vi "Easy XML Editor.vi"() -> ()   [LabVIEW 2026, in "VILab.lvlib"]
doc: "A tool for editing LabVIEW objects as XML that's quicker than using the other resource editor VI."
uses:
  VILab.lvlib
  CTLs/XML Editor State Data.ctl
  CTLs/Resource.ctl
  <vilib>/Utility/miscctls.llb/LVPositionTypeDef.ctl
  <vilib>/ErrorRing/Error Ring.xnode
  SubVIs/FaKI State Machine/FaKI State Machine.lvlib
panel:
  in  "Exit":bool
  in  "Paste FP":bool
  in  "Copy FP":bool
  in  "Front Panel XML/VTT":string
  in  "Paste BD":bool
  in  "Copy BD":bool
  in  "Block Diagram XML/VTT":string
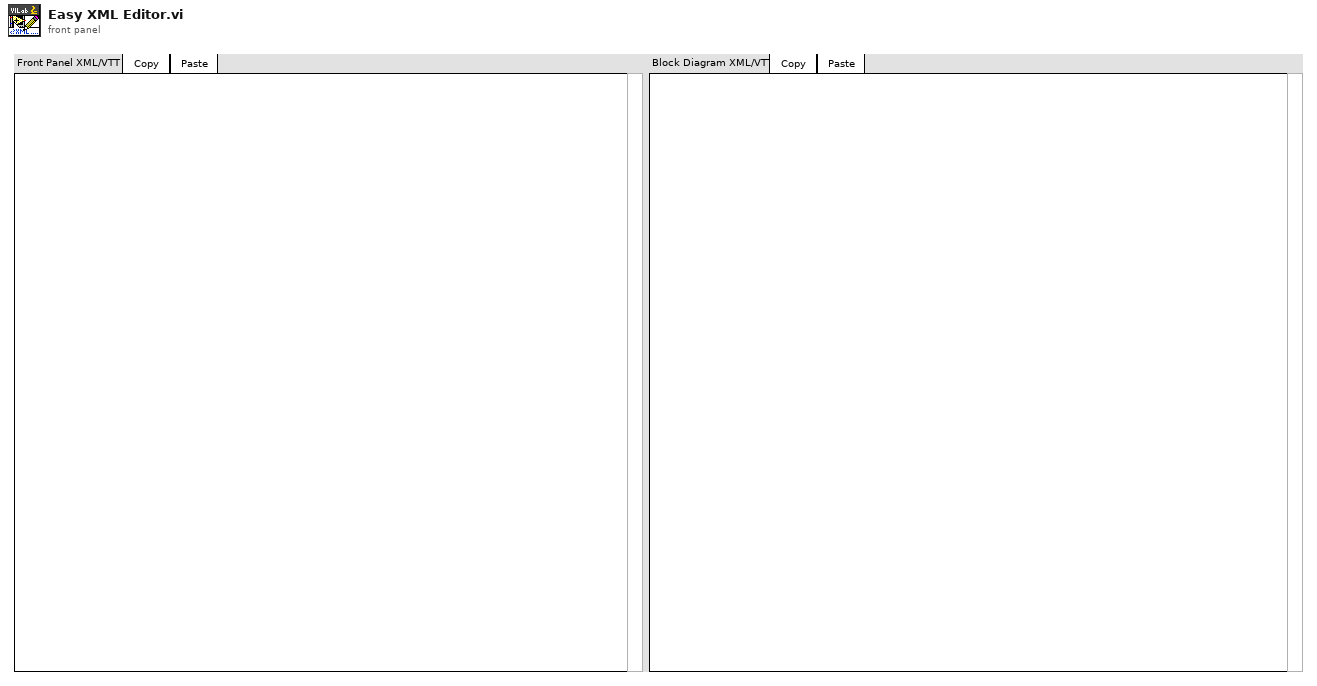
[diagram p1: front panel]
types:
  T1 = typedef "VILab.lvlib/XML Editor State Data.ctl" = cluster{"Core":cluster{"Current VI Ref":refnum<vi>, "Close Panel on Exit?":bool, "Menu Ref":refnum<k9>}, "Stored Resources":T2[], "Use Stored Resources?":bool, "Last Edited VI Path":path, "Use VTT?":bool, "Source VI Ref":refnum<vi>, "Booleans":cluster{"Refnum":refnum<vi>, "Position":T3}[], "FP XML":string, "BD XML":string}
  T2 = typedef "VILab.lvlib/Resource.ctl" = cluster{"type":u32, "id":i32, "name":string, "binary data":string}
  T3 = typedef "LVPositionTypeDef.ctl" = cluster{"Left":i32, "Top":i32}
  T4 = enum32{"Invalid", "Standard", "Closed", "Hidden", "Minimized", "Maximized"}
  T5 = enum32{"invalid app kind", "Development System", "Run Time System", "Student Edition", "Embedded LabVIEW", "Evaluation", "Custom"}
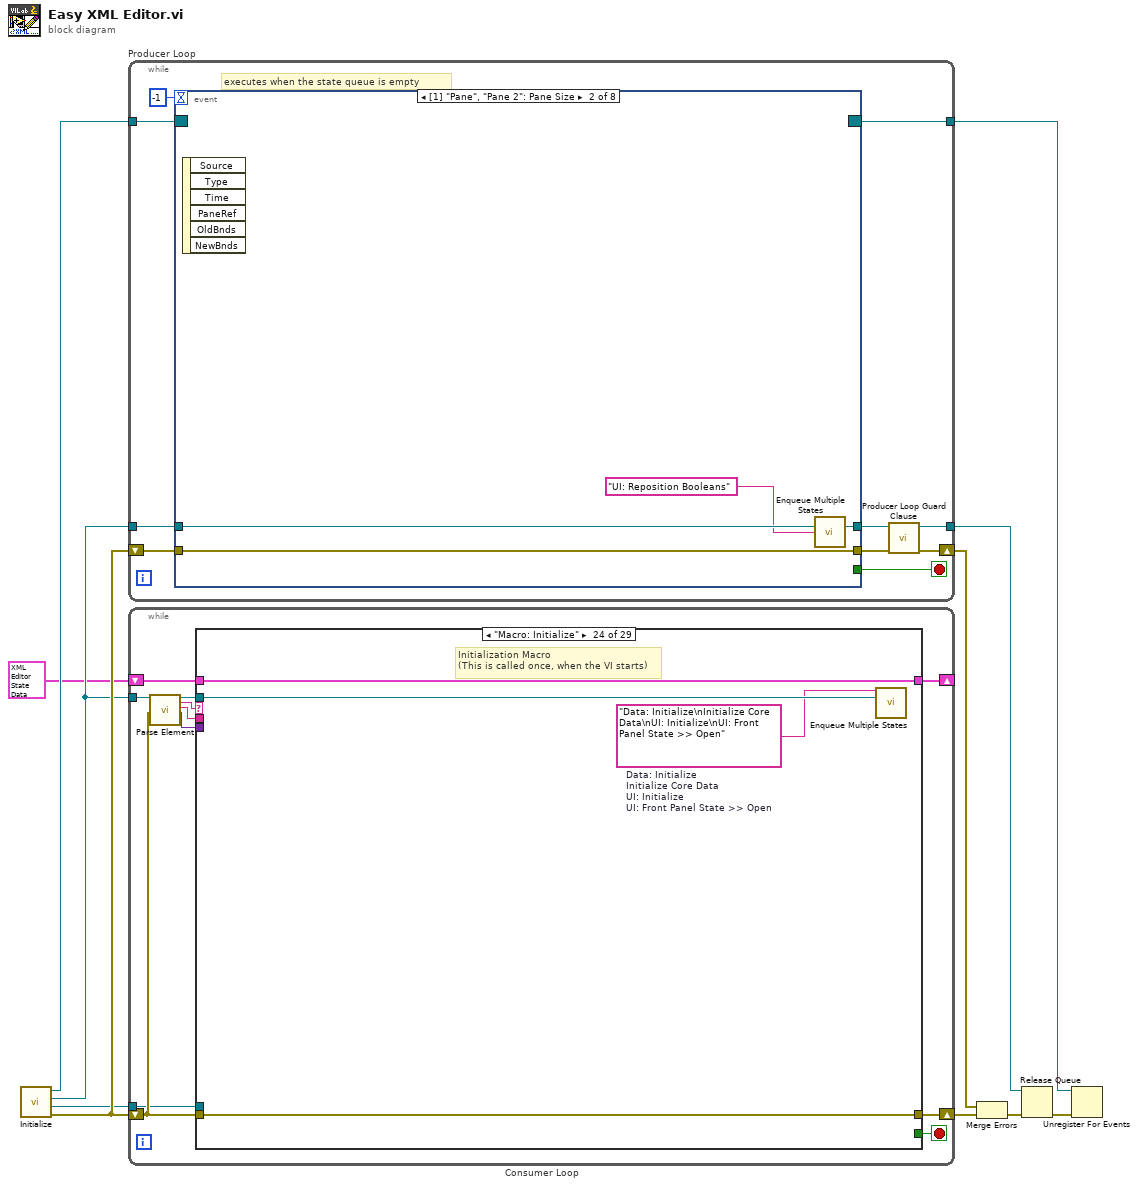
[diagram p0: block diagram]
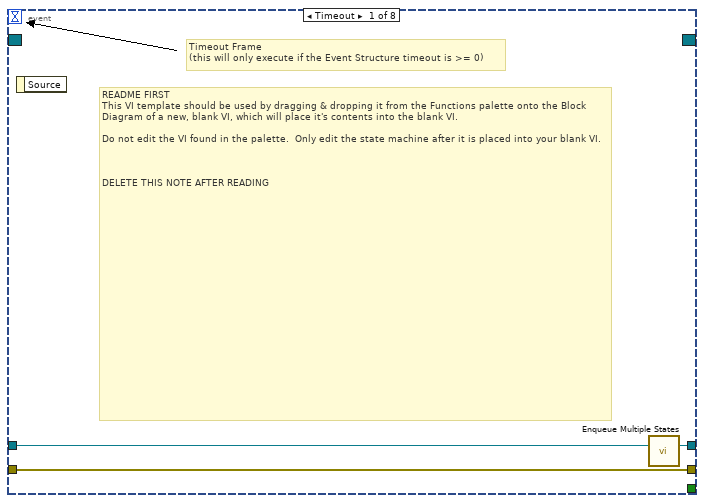
[diagram p2: hidden frame]
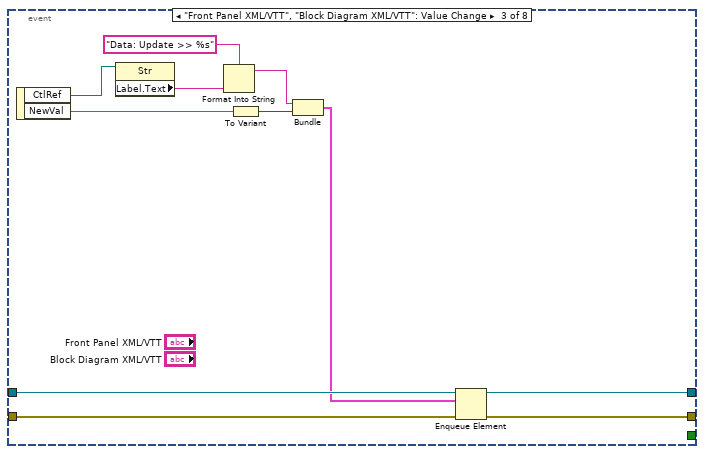
[diagram p3: hidden frame]
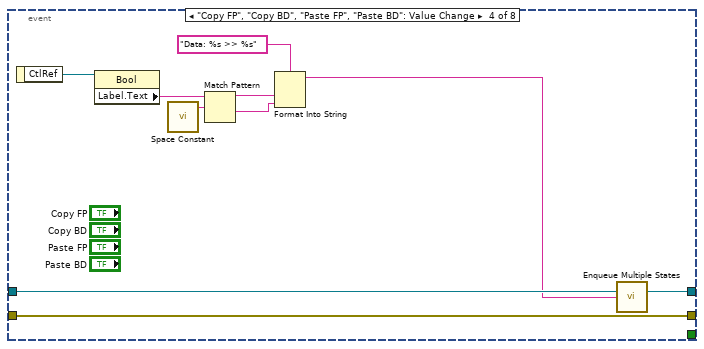
[diagram p4: hidden frame]
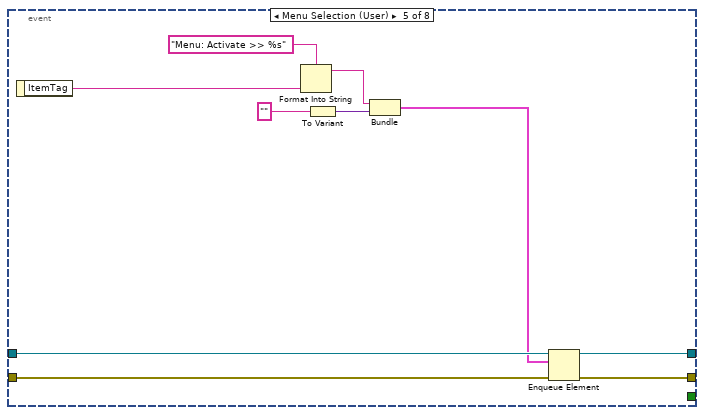
[diagram p5: hidden frame]
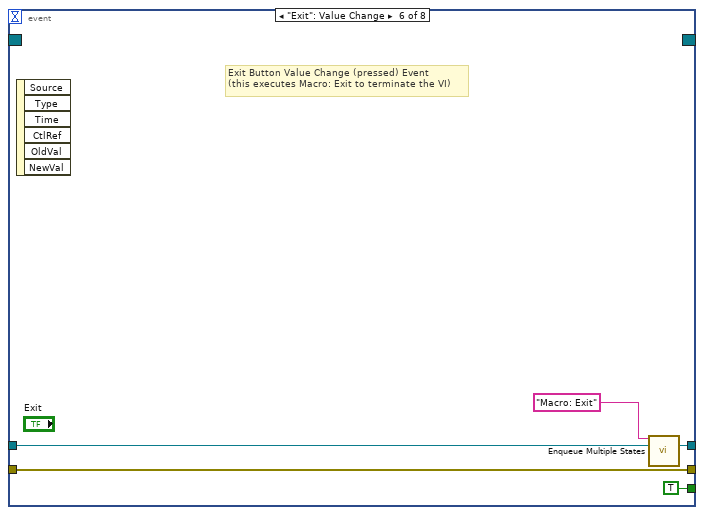
[diagram p6: hidden frame]
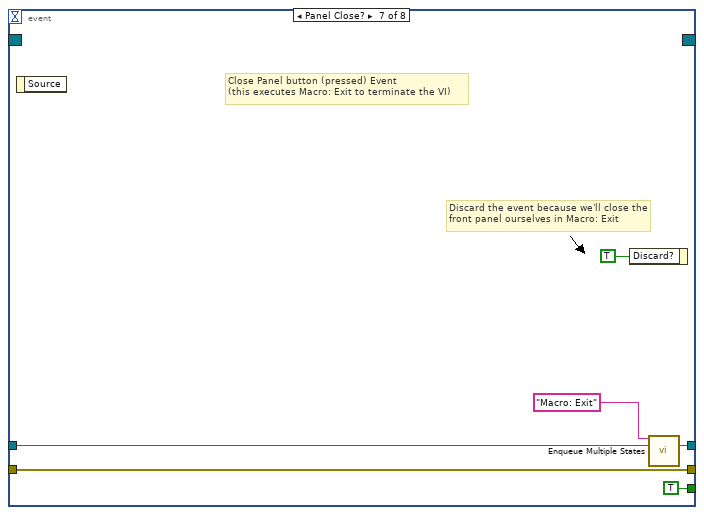
[diagram p7: hidden frame]
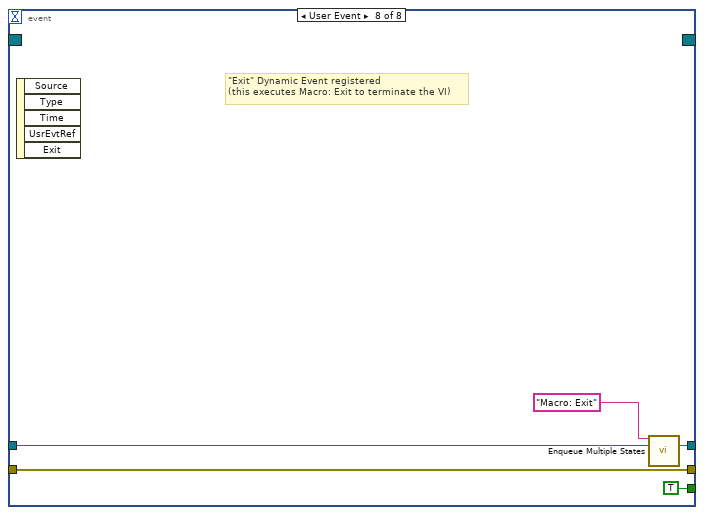
[diagram p8: hidden frame]
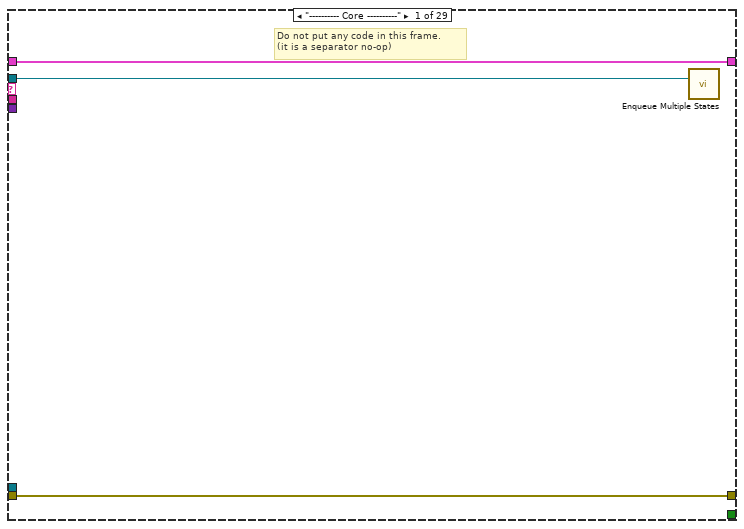
[diagram p9: hidden frame]
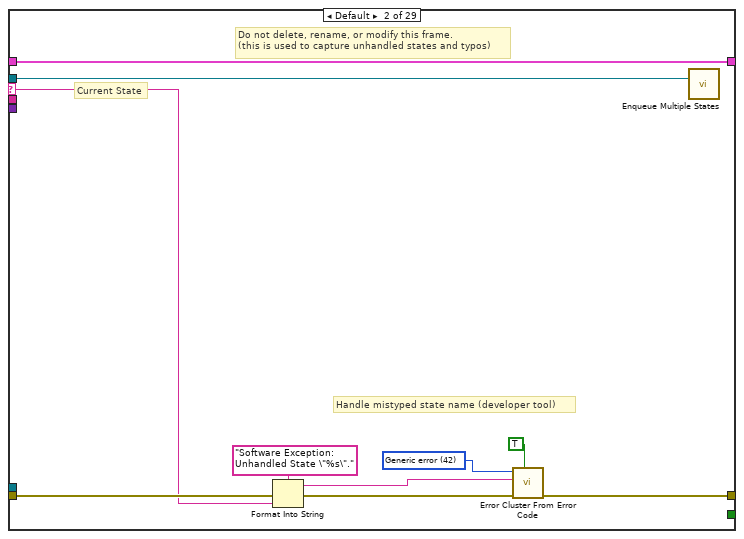
[diagram p10: hidden frame]
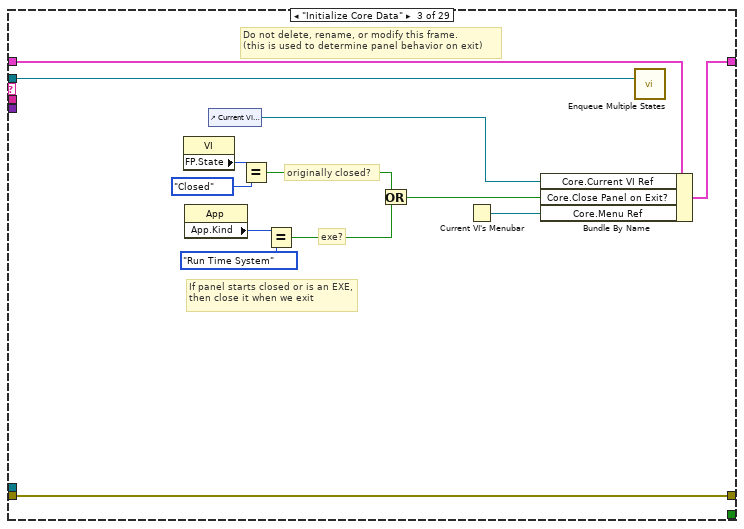
[diagram p11: hidden frame]
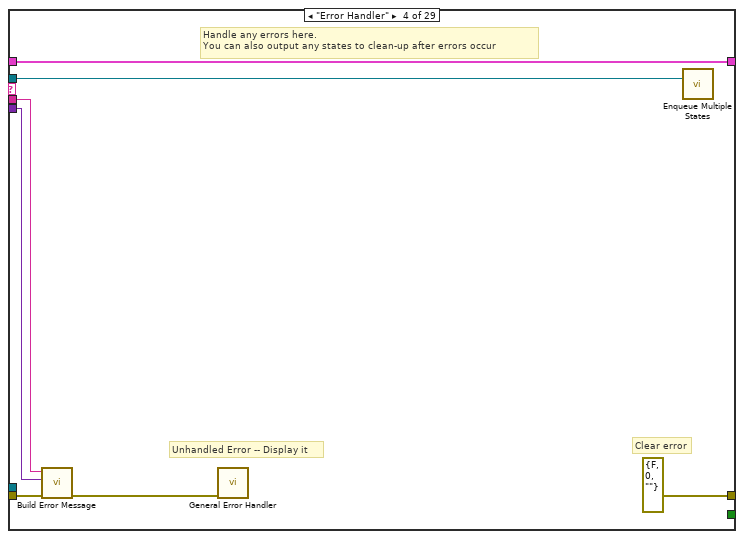
[diagram p12: hidden frame]
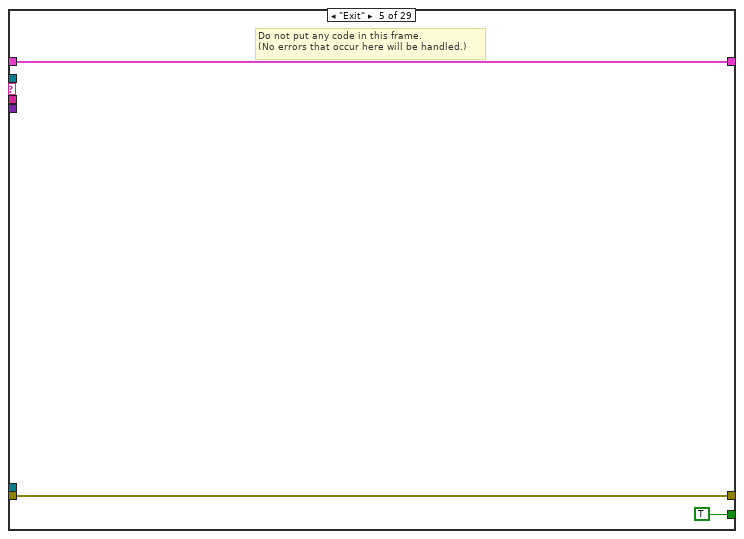
[diagram p13: hidden frame]
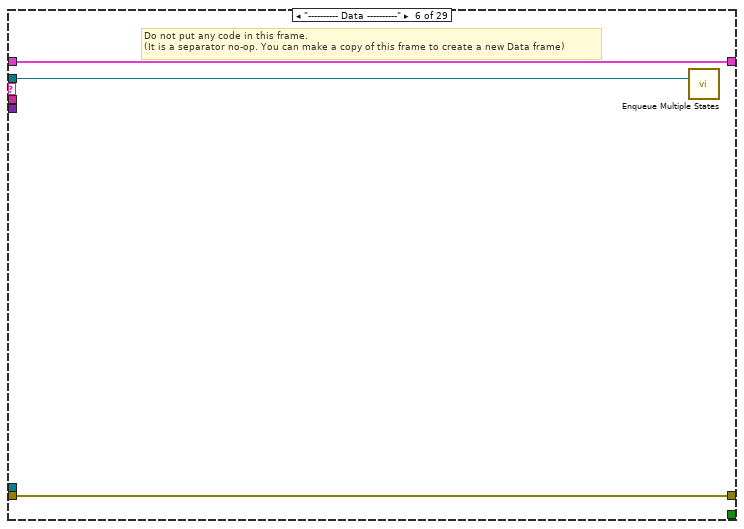
[diagram p14: hidden frame]
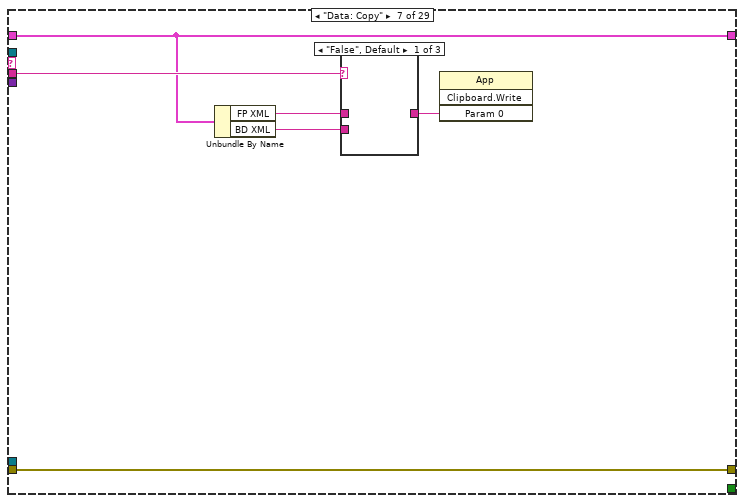
[diagram p15: hidden frame]
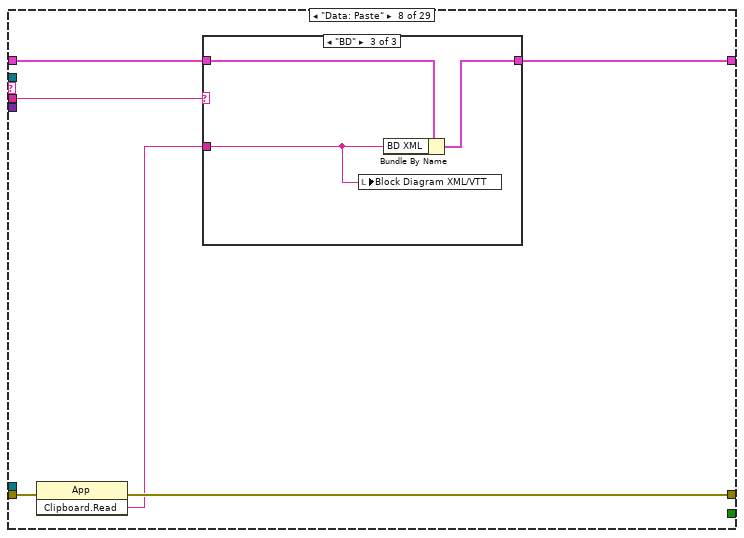
[diagram p18: hidden frame]
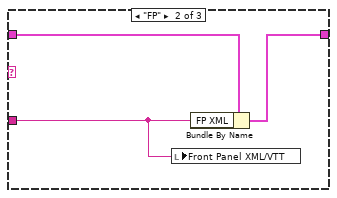
[diagram p20: hidden frame]
diagram:
  n1 = call "Initialize.vi"() -> ("error out"=w7:errorcluster, "Exit Event out"=w4:refnum<user-event>, "queue out"=w6:refnum<queue>, "Event Registration Refnum out"=w5:refnum<event-registration>)  [unwired: 8 in]
  n2 = while "Producer Loop" {
    shift-right: [w16] -> w10
    shift-left: w7 -> [w21]
    tunnel: w5 -> [w13]
    tunnel: w6 -> [w19]
    tunnel: [w14] -> w8
    tunnel: [w12] -> w2
    stop <- w18 stop-if-true
    # "executes when the state queue is empty"
    n3 = event shown="[1] \"Pane\", \"Pane 2\": Pane Size" {
      selector: w13 -> [_ _ _ _ _ _ _ _]
      dyn-events: [_ _ _ _ _ _ _ _] -> w12
      timeout: -1 ("Timeout") -> [_ _ _ _ _ _ _ _]
      tunnel: [w22 w26 w38 w49 w58 w64 w70 w75] -> w17
      tunnel: w21 -> [w22 w26 w39 w49 w59 w64 w70 w75]
      tunnel: w19 -> [w23 w27 w37 w48 w57 w63 w67 w73]
      tunnel: [w24 w28 w36 w47 w56 w61 w66 w72] -> w15
      tunnel: [_ _ _ _ _ TRUE TRUE TRUE] -> w18
      event Timeout {
        # "README FIRST\nThis VI template should be used by dragging & dropping it from the Functions palette onto the Block Diagram of a new, blank VI, which will place it's contents into the blank VI.\n\nDo not edit the VI found in the palette.  Only edit the state machine after it is placed into your blank VI.\n\n\n\nDELETE THIS NOTE AFTER READING"
        # "Timeout Frame\n(this will only execute if the Event Structure timeout is >= 0)"
        n4 = event-data() -> ()  [unwired: 1 in, 1 out]
        n5 = call "Enqueue Multiple States.vi"("queue in"=w23) -> ("queue out"=w24:refnum<queue>)  [unwired: 14 in]
      }
      event Pane Size {
        n6 = event-data() -> ()  [unwired: 1 in, 6 out]
        n7 = call "Enqueue Multiple States.vi"("queue in"=w27, "State(s) at Back"="UI: Reposition Booleans") -> ("queue out"=w28:refnum<queue>)  [unwired: 13 in]
      }
      event "Front Panel XML/VTT", "Block Diagram XML/VTT": Value Change {
        n8 = event-data() -> ("CtlRef"=w35:refnum<vi>, "NewVal"=w32:string)  [unwired: 1 in]
        n9 = property class="Str"(reference=w35) -> ("Label.Text"=w33:string)  [unwired: 1 in, 2 out]
        n10 = Format Into String(format string="Data: Update >> %s", w33) -> (resulting string=w30:string)  [unwired: 2 in, 1 out]
        n11 = To Variant(anything=w32) -> (Variant=w31:variant)
        n12 = Bundle(w30, "Variant"=w31) -> (w29:cluster{string, "Variant":variant})  [unwired: 1 in]
        n13 = Enqueue Element(queue=w37, element=w29, error in (no error)=w39) -> (queue out=w36:refnum<queue>, error out=w38:errorcluster)  [unwired: 1 in, 1 out]
      }
      event "Copy FP", "Copy BD", "Paste FP", "Paste BD": Value Change {
        n14 = event-data() -> ("CtlRef"=w46:refnum<vi>)  [unwired: 1 in]
        n15 = property class="Bool"(reference=w46) -> ("Label.Text"=w44:string)  [unwired: 1 in, 2 out]
        n16 = call <vilib>:"Space Constant.vi"() -> ("String"=w43:string)
        n17 = Match Pattern(string=w44, regular expression=w43) -> (before substring=w42:string, after substring=w41:string)  [unwired: 1 in, 2 out]
        n18 = Format Into String(format string="Data: %s >> %s", w42, w41) -> (resulting string=w40:string)  [unwired: 2 in, 1 out]
        n19 = call "Enqueue Multiple States.vi"("queue in"=w48, "State(s) at Back"=w40) -> ("queue out"=w47:refnum<queue>)  [unwired: 13 in]
      }
      event Menu Selection (User) {
        n20 = event-data() -> ("ItemTag"=w50:string)  [unwired: 1 in]
        n21 = Format Into String(format string="Menu: Activate >> %s", w50) -> (resulting string=w53:string)  [unwired: 2 in, 1 out]
        n22 = To Variant(anything="") -> (Variant=w54:variant)
        n23 = Bundle(w53, "Variant"=w54) -> (w52:cluster{string, "Variant":variant})  [unwired: 1 in]
        n24 = Enqueue Element(queue=w57, element=w52, error in (no error)=w59) -> (queue out=w56:refnum<queue>, error out=w58:errorcluster)  [unwired: 1 in, 1 out]
      }
      event "Exit": Value Change {
        # "Exit Button Value Change (pressed) Event\n(this executes Macro: Exit to terminate the VI)"
        n25 = event-data() -> ()  [unwired: 1 in, 6 out]
        n26 = call "Enqueue Multiple States.vi"("State(s) at Front"="Macro: Exit", "queue in"=w63) -> ("queue out"=w61:refnum<queue>)  [unwired: 13 in]
      }
      event Panel Close? {
        # "Discard the event because we'll close the front panel ourselves in Macro: Exit"
        # "Close Panel button (pressed) Event\n(this executes Macro: Exit to terminate the VI)"
        n27 = event-data() -> ()  [unwired: 1 in, 1 out]
        n28 = event-data("Discard?"=TRUE) -> ()  [unwired: 1 in, 1 out]
        n29 = call "Enqueue Multiple States.vi"("State(s) at Front"="Macro: Exit", "queue in"=w67) -> ("queue out"=w66:refnum<queue>)  [unwired: 13 in]
      }
      event User Event {
        # "\"Exit\" Dynamic Event registered\n(this executes Macro: Exit to terminate the VI)"
        n30 = event-data() -> ()  [unwired: 1 in, 5 out]
        n31 = call "Enqueue Multiple States.vi"("State(s) at Front"="Macro: Exit", "queue in"=w73) -> ("queue out"=w72:refnum<queue>)  [unwired: 13 in]
      }
    }
    n32 = call "Producer Loop Guard Clause.vi"("error in (no error)"=w17, "queue in"=w15) -> ("error out"=w16:errorcluster, "queue out"=w14:refnum<queue>)  [unwired: 8 in]
  }
  n33 = while "Consumer Loop" {
    shift-right: [w83] -> _
    shift-left: T1 {"Core"={"Current VI Ref"=refnum, "Close Panel on Exit?"=FALSE, "Menu Ref"=refnum}, "Stored Resources"=[], "Use Stored Resources?"=TRUE, "Last Edited VI Path"=path "", "Use VTT?"=FALSE, "Source VI Ref"=refnum, "Booleans"=[], "FP XML"="", "BD XML"=""} ("XML Editor State Data") -> [w82]
    shift-right: [w86] -> w11
    shift-left: w7 -> [w85]
    tunnel: w6 -> [w81]
    tunnel: w4 -> [w76]
    stop <- w84 stop-if-true
    n34 = call "Parse Element.vi"("queue in"=w81, "error in (no error)"=w85) -> ("queue out"=w80:refnum<queue>, "State"=w79:string, "Arg"=w78:string, "Data"=w77:variant)  [unwired: 14 in]
    n35 = case shown="\"Macro: Initialize\"" w79 {
      selector: w79 -> [_ w91 _ _ _ _ _ _ _ _ _ _ _ _ _ _ _ _ _ _ _ _ _ _ _ _ _ _ _]
      tunnel: w80 -> [w87 w90 w101 w117 _ w123 _ _ _ _ _ _ w239 w243 _ _ _ _ _ w282 w285 w294 w365 w369 w375 w381 _ w390 _]
      tunnel: w78 -> [_ _ _ w113 _ _ w130 w139 _ w164 _ _ _ _ _ _ _ _ _ _ w286 w295 _ _ _ _ _ w389 w421]
      tunnel: w82 -> [w88 w93 w107 w118 w121 w124 w129 w136 w149 w163 w204 w219 w240 w244 w248 w257 w266 w272 w276 w283 w287 w297 w366 w370 w379 w382 w385 w391 w418]
      tunnel: [w89 w98 w112 errorcluster {"status"=FALSE, "code"=0, "source"=""} ("error out") w122 w125 w131 w137 w155 w160 w207 w220 w242 w245 w249 w260 w262 w270 w277 w284 w288 w298 w367 w371 w380 w383 w386 w392 w419] -> w86
      tunnel: w85 -> [w89 w97 w112 w116 w122 w125 w131 w138 w155 w165 w208 w213 w238 w245 w250 w260 w263 w270 w277 w284 w289 w299 w367 w371 w380 w383 w387 w392 w420]
      tunnel: [_ _ _ _ TRUE _ _ _ _ _ _ _ _ _ _ _ _ _ _ _ _ _ _ _ _ _ _ _ _] -> w84
      tunnel: [w88 w93 w111 w118 w121 w124 w129 w135 w147 w161 w202 w218 w240 w244 w247 w257 w266 w271 w276 w283 w287 w297 w366 w370 w379 w382 w385 w391 w418] -> w83
      tunnel: w77 -> [_ _ _ w114 _ _ _ _ _ w162 _ _ _ _ _ _ _ _ _ _ _ _ _ _ _ _ _ _ _]
      tunnel: w76 -> [_ _ _ _ _ _ _ _ _ _ _ _ w237 _ _ _ _ _ _ _ _ _ _ _ _ _ _ _ _]
      frame "---------- Core ----------" {
        # "Do not put any code in this frame.\n(it is a separator no-op)"
        n36 = call "Enqueue Multiple States.vi"("queue in"=w87) -> ()  [unwired: 14 in, 1 out]
      }
      frame Default {
        w95 = 42 items=["No error", "Argument error", "Memory is full", "Out of zone", "End of file", "File already open", "Generic file I/O error", "File not found", "File permission error", "Disk is full", "Duplicate path", "Too many files open", "System feature not enabled", "Resource file not found", "Cannot add resource", "Resource not found", "Image not found", "Image memory error", "Pen does not exist", "Config type invalid", "Config token not found", "Config parse error", "Config memory error", "Bad external code format", "Bad external code offset", "External code not present", "Null window", "Destroy window error", "Null menu", "Print aborted", "Bad print record", "Print driver error", "Windows error during printing", "Memory error during printing", "Print dialog error", "Generic print error", "Invalid device refnum", "Device not found", "Device parameter error", "Device unit error", "Cannot open device", "Device call aborted", "Generic error", "Cancelled by user", "Object ID too low", "Object ID too high", "Object not in heap", "Unknown heap", "Unknown object (invalid DefProc)", "Unknown object (DefProc not in table)", "Message out of range", "Invalid (null) method", "Unknown message", "Manager call not supported", "Bad address", "Network operation in progress", "Network operation timed out", "Connection is busy", "Network attribute not supported", "Network error", "Address in use", "System out of memory", "Connection aborted", "Connection refused", "Not connected", "Already connected", "Connection closed", "Initialization error (interapplication manager)", "Bad occurrence", "Wait on unbound occurrence handler", "Occurrence queue overflow", "Datalog type conflict", "Unused", "Unrecognized type (interapplication manager)", "Memory corrupt", "Failed to make temporary DLL", "Old CIN version", "Drag socket not found", "Failed to load drop-object", "Failed to register OLE object", "Failed to release OLE object", "Format specifier type mismatch", "Unknown format specifier", "Too few format specifiers", "Too many format specifiers", "Scan failed", "Newer CIN version", "Error converting to variant", "Runtime menu error", "Password tampered", "Variant attribute not found", "Incompatible variant data type", "Event data is not available", "Event Store is not present", "Occurrence is not found", "Event Queue is not created", "Event info is not available", "Refnum passed is NULL", "Error retrieving Class GUID", "Error retrieving CoClass GUID", "Error retrieving TypeLib GUID.", "Bad built application magic bytes.", "Specific driver is different from the specific driver associated with the Logical Name.", "There is no session opened to the class driver.", "Max Error", "MAX - Error with config objects", "MAX - Error loading configuration", "MAX - Group not supported"]
        # "Current State"
        # "Do not delete, rename, or modify this frame.\n(this is used to capture unhandled states and typos)"
        # "Handle mistyped state name (developer tool)"
        n37 = Format Into String(format string="Software Exception: Unhandled State \"%s\"." ("message"), error in=w97, w91) -> (resulting string=w94:string, error out=w99:errorcluster)  [unwired: 1 in]
        n38 = call <vilib>:"Error Cluster From Error Code.vi"("show call chain? (False)"=TRUE, "error in (no error)"=w99, "error message (\"\")"=w94, "error code (0)"=w95) -> ("error out"=w98:errorcluster)  [unwired: 5 in]
        n39 = call "Enqueue Multiple States.vi"("queue in"=w90) -> ()  [unwired: 14 in, 1 out]
      }
      frame "Initialize Core Data" {
        # "Do not delete, rename, or modify this frame.\n(this is used to determine panel behavior on exit)"
        # "originally closed?"
        # "exe?"
        # "If panel starts closed or is an EXE, then close it when we exit"
        n40 = property class="VI"() -> ("FP.State"=w104:T4)  [unwired: 2 in, 2 out]
        n41 = property class="App"() -> ("App.Kind"=w110:T5)  [unwired: 2 in, 2 out]
        n42 = control-ref of="Current VI Reference"() -> (w105:refnum<vi>)
        n43 = Equal?(x=w104, y=T4."Closed" ("Front Panel Window:State")) -> (x = y?=w102:bool)
        n44 = Equal?(x=w110, y=T5."Run Time System" ("Application:Kind")) -> (x = y?=w108:bool)
        n45 = Or(x=w102, y=w108) -> (x .or. y?=w106:bool)
        n46 = Current VI's Menubar() -> (w100:refnum<k9>)
        n47 = Bundle By Name(cluster=w107, "Core.Current VI Ref"=w105, "Core.Close Panel on Exit?"=w106, "Core.Menu Ref"=w100) -> (w111:T1)
        n48 = call "Enqueue Multiple States.vi"("queue in"=w101) -> ()  [unwired: 14 in, 1 out]
      }
      frame "Error Handler" {
        # "Unhandled Error -- Display it"
        # "Handle any errors here.\nYou can also output any states to clean-up after errors occur"
        # "Clear error"
        n49 = call "Build Error Message.vi"("error in (no error)"=w116, "Data"=w114, "Arg"=w113) -> ("error out"=w115:errorcluster)  [unwired: 8 in]
        n50 = call <vilib>:"General Error Handler.vi"("error in (no error)"=w115) -> ()  [unwired: 10 in, 5 out]
        n51 = call "Enqueue Multiple States.vi"("queue in"=w117) -> ()  [unwired: 14 in, 1 out]
      }
      frame "Exit" {
        # "Do not put any code in this frame.\n(No errors that occur here will be handled.)"
      }
      frame "---------- Data ----------" {
        # "Do not put any code in this frame.\n(It is a separator no-op. You can make a copy of this frame to create a new Data frame)"
        n52 = call "Enqueue Multiple States.vi"("queue in"=w123) -> ()  [unwired: 14 in, 1 out]
      }
      frame "Data: Copy" {
        n53 = Unbundle By Name(w129) -> ("FP XML"=w128:string, "BD XML"=w126:string)
        n54 = case shown="\"False\", Default" w130 {
          tunnel: w128 -> [_ w132 _]
          tunnel: [_ w132 w133] -> w127
          tunnel: w126 -> [_ _ w133]
          frame "False", Default {
          }
          frame "FP" {
          }
          frame "BD" {
          }
        }
        n55 = invoke class="App" method="Clipboard.Write"("Param 0"=w127) -> ()  [unwired: 3 in, 4 out]
      }
      frame "Data: Paste" {
        n56 = invoke class="App" method="Clipboard.Read"(error in=w138) -> (error out=w137:errorcluster, "Read Clipbrd"=w134:string)  [unwired: 2 in, 1 out]
        n57 = case shown="\"BD\"" w139 {
          tunnel: w136 -> [w140 w143 w146]
          tunnel: [w140 w142 w145] -> w135
          tunnel: w134 -> [_ w141 w144]
          frame "False", Default {
          }
          frame "FP" {
            n58 = local write "Front Panel XML/VTT"(w141) -> ()
            n59 = Bundle By Name(cluster=w143, "FP XML"=w141) -> (w142:T1)
          }
          frame "BD" {
            n60 = local write "Block Diagram XML/VTT"(w144) -> ()
            n61 = Bundle By Name(cluster=w146, "BD XML"=w144) -> (w145:T1)
          }
        }
      }
      frame "Data: Initialize" {
        # "Initialize the shift-register data, here."
        n62 = control-ref of="Copy FP"() -> (w150:refnum<vi>)
        n63 = control-ref of="Paste FP"() -> (w151:refnum<vi>)
        n64 = control-ref of="Copy BD"() -> (w152:refnum<vi>)
        n65 = control-ref of="Paste BD"() -> (w153:refnum<vi>)
        n66 = Build Array(w150, w151, w152, w153) -> (w154:refnum<vi>[])
        n67 = for {
          tunnel: w154 -> [w159] mode=indexing
          tunnel: [w156] -> w148 mode=indexing
          n68 = property class="Bool"(reference=w159) -> (reference out=w158:refnum<vi>, "Position"=w157:T3)  [unwired: 1 in, 1 out]
          n69 = Bundle("Paste BD"=w158, "Position"=w157) -> (w156:cluster{"Paste BD":refnum<vi>, "Position":T3})  [unwired: 1 in]
        }
        n70 = Bundle By Name(cluster=w149, "Booleans"=w148) -> (w147:T1)
      }
      frame "Data: Update" {
        n71 = case shown="Default" w164 {
          selector: w164 -> [w167 _ _ _ _]
          tunnel: w165 -> [_ w182 w189 w192 w197]
          tunnel: w163 -> [w168 w179 w186 w191 w196]
          tunnel: w162 -> [_ w180 w187 _ _]
          tunnel: [w168 w178 w185 w190 w195] -> w161
          tunnel: [w166 w177 w184 w192 w197] -> w160
          frame Default {
            n72 = xnode "Error Ring"("parameter 0"=w167) -> ("error out"=w166:errorcluster)
          }
          frame "Front Panel XML/VTT" {
            n73 = Variant To Data(error in=w182, type="", Variant=w180) -> (data=w176:string, error out=w177:errorcluster)
            n74 = Bundle By Name(cluster=w179, "FP XML"=w176) -> (w178:T1)
          }
          frame "Block Diagram XML/VTT" {
            n75 = Variant To Data(error in=w189, type="", Variant=w187) -> (data=w183:string, error out=w184:errorcluster)
            n76 = Bundle By Name(cluster=w186, "BD XML"=w183) -> (w185:T1)
          }
          frame "Use VTT?" {
            n77 = in-place {
              n78 = in-place-cluster #1(w191) -> ("Use VTT?"=w194:bool)
              n79 = Not(x=w194) -> (.not. x?=w193:bool)
              n80 = in-place-cluster #1("Use VTT?"=w193) -> (w190:T1)
            }
          }
          frame "Use Stored Resources?" {
            n81 = in-place {
              n82 = in-place-cluster #2(w196) -> ("Use Stored Resources?"=w199:bool)
              n83 = Not(x=w199) -> (.not. x?=w198:bool)
              n84 = in-place-cluster #2("Use Stored Resources?"=w198) -> (w195:T1)
            }
          }
        }
      }
      frame "Data: Source VI to Res Data" {
        n85 = Unbundle By Name(w204) -> ("Source VI Ref"=w206:refnum<vi>, "Use VTT?"=w205:bool)
        n86 = call "Convert Source VI to Resource Data.vi"("error in (no error)"=w208, "Use VTT?"=w205, "Source VI Ref"=w206) -> ("error out"=w207:errorcluster, "BD Resource Data"=w200:string, "FP Resource Data"=w201:string, "Resources"=w203:T2[])  [unwired: 5 in]
        n87 = Bundle By Name(cluster=w204, "Stored Resources"=w203, "FP XML"=w201, "BD XML"=w200) -> (w202:T1)
        n88 = local write "Front Panel XML/VTT"(w201) -> ()
        n89 = local write "Block Diagram XML/VTT"(w200) -> ()
      }
      frame "Data: Save VI from Res Data" {
        n90 = Unbundle By Name(w219) -> ("Use VTT?"=w217:bool, "FP XML"=w216:string, "BD XML"=w215:string, "Use Stored Resources?"=w211:bool, "Stored Resources"=w212:T2[])
        n91 = case shown="False" w211 {
          tunnel: [w227 w231] -> w209
          tunnel: w212 -> [_ w231]
          tunnel: w213 -> [w225 w230]
          tunnel: [w221 w230] -> w210
          frame False {
            n92 = New VI(8:w225) -> (0:w226:errorcluster, 3:w229:refnum<vi>)  [unwired: 6 in]
            n93 = call "Save VI with XML Heaps.vi"("error in (no error)"=w226, "VI Refnum In"=w229) -> ("error out"=w224:errorcluster, "VI Path out"=w228:path, "VI Refnum Out"=w222:refnum<vi>)  [unwired: 7 in]
            n94 = call "Load Resource File.vi"("error in (no error)"=w224, "Resource File"=w228) -> ("error out"=w223:errorcluster, "Resources"=w227:T2[])  [unwired: 7 in, 1 out]
            n95 = Close Reference(reference=w222, error in (no error)=w223) -> (error out=w221:errorcluster)
          }
          frame True {
          }
        }
        n96 = call "Save New VI From XML.vi"("Use VTT?"=w217, "error in (no error)"=w210, "Block Diagram XML/VTT"=w215, "Front Panel XML/VTT"=w216, "Resources"=w209) -> ("error out"=w220:errorcluster, "Unique Temporary File Path"=w214:path)  [unwired: 5 in]
        n97 = Bundle By Name(cluster=w219, "Last Edited VI Path"=w214) -> (w218:T1)
      }
      frame "Data: Cleanup" {
        # "\"already closed\" error"
        # "Cleanup any data and references, here.\n(this is called automatically, by the Macro: Exit)"
        n98 = Destroy User Event(user event=w237, error in=w238) -> (error out=w236:errorcluster)
        n99 = Unbundle By Name(w240) -> ("Source VI Ref"=w232:refnum<vi>, "Core.Current VI Ref"=w241:refnum<vi>)
        n100 = Close Reference(reference=w241, error in (no error)=w236) -> (error out=w242:errorcluster)
        n101 = invoke class="VI" method="FP.Close"(reference=w232) -> (reference out=w235:refnum<vi>, error out=w234:errorcluster)  [unwired: 2 in, 1 out]
        n102 = Close Reference(reference=w235) -> ()  [unwired: 1 in, 1 out]
        n103 = call <vilib>:"Clear Errors.vi"("error in (no error)"=w234, "specific error code to clear (0: all)"=1149) -> ()  [unwired: 4 in, 2 out]
        n104 = call "Enqueue Multiple States.vi"("queue in"=w239) -> ()  [unwired: 14 in, 1 out]
      }
      frame "---------- UI ----------" {
        # "Do not put any code in this frame.\n(It is a separator no-op. You can make a copy of this frame to create a new UI frame)"
        n105 = call "Enqueue Multiple States.vi"("queue in"=w243) -> ()  [unwired: 14 in, 1 out]
      }
      frame "UI: Open Source VI" {
        n106 = New VI(8:w250) -> (0:w252:errorcluster, 3:w255:refnum<vi>)  [unwired: 6 in]
        n107 = invoke class="VI" method="FP.Open"(reference=w255, error in=w252) -> (reference out=w256:refnum<vi>, error out=w251:errorcluster)  [unwired: 3 in, 3 out]
        n108 = property class="VI"(reference=w256, error in=w251, "BDWin.Open"=TRUE ("Block Diagram Window:Open"), "Front Panel.Title"="Source VI") -> (reference out=w246:refnum<vi>, error out=w249:errorcluster)
        n109 = Bundle By Name(cluster=w248, "Source VI Ref"=w246) -> (w247:T1)
      }
      frame "UI: Resource Editor" {
        n110 = Unbundle By Name(w257) -> ("Last Edited VI Path"=w259:path)
        n111 = call "Resource Editor--Legacy.vi"("Load from Initial Path (F)"=TRUE, "Path"=w259) -> ()  [unwired: 9 in, 1 out]
      }
      frame "UI: Open Edited VI" {
        n112 = Unbundle By Name(w266) -> ("Last Edited VI Path"=w269:path)
        n113 = Open VI Reference(vi path=w269, error in (no error)=w263) -> (vi reference=w268:refnum<vi>, error out=w265:errorcluster)  [unwired: 4 in]
        n114 = invoke class="VI" method="FP.Open"(reference=w268, error in=w265, "Activate"=TRUE ("Activate?")) -> (reference out=w267:refnum<vi>, error out=w264:errorcluster)  [unwired: 2 in, 3 out]
        n115 = Close Reference(reference=w267, error in (no error)=w264) -> (error out=w262:errorcluster)
      }
      frame "UI: Edit Stored Resources" {
        n116 = in-place {
          n117 = in-place-cluster #3(w272) -> ("Stored Resources"=w274:T2[])
          n118 = call "Resource Editor--Legacy.vi"("Initial Resources"=w274) -> ("Final Resources"=w273:T2[])  [unwired: 10 in]
          n119 = in-place-cluster #3("Stored Resources"=w273) -> (w271:T1)
        }
      }
      frame "UI: Reposition Booleans" {
        n120 = Unbundle By Name(w276) -> ("Booleans"=w275:cluster{"Refnum":refnum<vi>, "Position":T3}[])
        n121 = for {
          tunnel: w275 -> [w280] mode=indexing
          n122 = Unbundle(w280) -> ("Refnum"=w279:refnum<vi>, "Position"=w278:T3)
          n123 = property class="Bool"(reference=w279, "Position"=w278) -> ()  [unwired: 1 in, 2 out]
        }
      }
      frame "UI: Initialize" {
        # "Initialize the User Interface, here.\n(this is called automatically, by the Macro: Init)"
        n124 = call "Enqueue Multiple States.vi"("State(s) at Front"="Menu: Initialize\nUI: Open Source VI", "queue in"=w282) -> ()  [unwired: 13 in, 1 out]
      }
      frame "UI: Cursor Set" {
        # "Argument"
        # "Set and Unset Cursor Busy.\n(Usage: \"UI: Cursor Set >> Busy|Idle\")"
        n125 = case shown="\"Idle\", Default" w286 {
          tunnel: w289 -> [w291 w293]
          tunnel: [w290 w292] -> w288
          frame "Idle", Default {
            n126 = call <vilib>:"Unset Busy.vi"("error in (no error)"=w291) -> ("error out"=w290:errorcluster)  [unwired: 10 in]
          }
          frame "Busy" {
            n127 = call <vilib>:"Set Busy.vi"("error in (no error)"=w293) -> ("error out"=w292:errorcluster)  [unwired: 9 in, 1 out]
          }
        }
        n128 = call "Enqueue Multiple States.vi"("queue in"=w285) -> ()  [unwired: 14 in, 1 out]
      }
      frame "UI: Front Panel State" {
        # "Argument"
        # "Set Front Panel Open or Closed\n(Usage: \"UI: Front Panel State >> Open|Close\")"
        n129 = Unbundle By Name(w297) -> ("Core.Current VI Ref"=w296:refnum<vi>)
        n130 = case shown="\"Open\", \"Standard\", Default" w295 {
          tunnel: w299 -> [w306 w320 w332 w345 w358]
          tunnel: [w307 w321 w333 w346 w359] -> w298
          tunnel: w296 -> [w304 w318 w330 w343 w356]
          frame "Open", "Standard", Default {
            w300 = T4."Standard" ("State")
            n131 = property class="VI"(reference=w304, error in=w306) -> (reference out=w303:refnum<vi>, error out=w305:errorcluster, "FP.State"=w302:T4)
            n132 = Not Equal?(x=w302, y=w300) -> (x != y?=w301:bool)
            n133 = case shown="True" w301 {
              tunnel: [w312 w313] -> w307
              tunnel: w305 -> [w311 w313]
              tunnel: w303 -> [w309 _]
              tunnel: w300 -> [w308 _]
              frame True {
                n134 = invoke class="VI" method="FP.Open"(reference=w309, error in=w311, "Activate"=TRUE, "State"=w308) -> (error out=w312:errorcluster)  [unwired: 1 in, 4 out]
              }
              frame False {
              }
            }
          }
          frame "Close", "Closed" {
            n135 = property class="VI"(reference=w318, error in=w320) -> (reference out=w317:refnum<vi>, error out=w319:errorcluster, "FP.State"=w315:T4)
            n136 = Not Equal?(x=w315, y=T4."Closed" ("Front Panel Window:State")) -> (x != y?=w314:bool)
            n137 = case shown="True" w314 {
              tunnel: [w322 w325] -> w321
              tunnel: w319 -> [w322 w324]
              tunnel: w317 -> [_ w323]
              frame False {
              }
              frame True {
                n138 = invoke class="VI" method="FP.Close"(reference=w323, error in=w324) -> (error out=w325:errorcluster)  [unwired: 1 in, 2 out]
              }
            }
          }
          frame "Hidden", "Hide" {
            w326 = T4."Hidden" ("State")
            n139 = property class="VI"(reference=w330, error in=w332) -> (reference out=w329:refnum<vi>, error out=w331:errorcluster, "FP.State"=w328:T4)
            n140 = Not Equal?(x=w328, y=w326) -> (x != y?=w327:bool)
            n141 = case shown="True" w327 {
              tunnel: [w337 w338] -> w333
              tunnel: w331 -> [w336 w338]
              tunnel: w329 -> [w335 _]
              tunnel: w326 -> [w334 _]
              frame True {
                n142 = invoke class="VI" method="FP.Open"(reference=w335, error in=w336, "State"=w334) -> (error out=w337:errorcluster)  [unwired: 2 in, 4 out]
              }
              frame False {
              }
            }
          }
          frame "Minimize", "Minimized" {
            w339 = T4."Minimized" ("State")
            n143 = property class="VI"(reference=w343, error in=w345) -> (reference out=w342:refnum<vi>, error out=w344:errorcluster, "FP.State"=w341:T4)
            n144 = Not Equal?(x=w341, y=w339) -> (x != y?=w340:bool)
            n145 = case shown="True" w340 {
              tunnel: [w350 w351] -> w346
              tunnel: w344 -> [w349 w351]
              tunnel: w342 -> [w348 _]
              tunnel: w339 -> [w347 _]
              frame True {
                n146 = invoke class="VI" method="FP.Open"(reference=w348, error in=w349, "State"=w347) -> (error out=w350:errorcluster)  [unwired: 2 in, 4 out]
              }
              frame False {
              }
            }
          }
          frame "Maximize", "Maximized" {
            w352 = T4."Maximized" ("State")
            n147 = property class="VI"(reference=w356, error in=w358) -> (reference out=w355:refnum<vi>, error out=w357:errorcluster, "FP.State"=w354:T4)
            n148 = Not Equal?(x=w354, y=w352) -> (x != y?=w353:bool)
            n149 = case shown="True" w353 {
              tunnel: [w363 w364] -> w359
              tunnel: w357 -> [w362 w364]
              tunnel: w355 -> [w361 _]
              tunnel: w352 -> [w360 _]
              frame True {
                n150 = invoke class="VI" method="FP.Open"(reference=w361, error in=w362, "State"=w360) -> (error out=w363:errorcluster)  [unwired: 2 in, 4 out]
              }
              frame False {
              }
            }
          }
        }
        n151 = call "Enqueue Multiple States.vi"("queue in"=w294) -> ()  [unwired: 14 in, 1 out]
      }
      frame "---------- Macro ----------" {
        # "Do not put any code in this frame.\n(It is a separator no-op. You can make a copy of this frame to create a new Macro frame)"
        n152 = call "Enqueue Multiple States.vi"("queue in"=w365) -> ()  [unwired: 14 in, 1 out]
      }
      frame "Macro: Initialize" {
        w368 = "Data: Initialize\nInitialize Core Data\nUI: Initialize\nUI: Front Panel State >> Open"  # Data: Initialize Initialize Core Data UI: Initialize UI: Front Panel State >> Open
        # "Initialization Macro\n(This is called once, when the VI starts)"
        n153 = call "Enqueue Multiple States.vi"("State(s) at Front"=w368, "queue in"=w369) -> ()  [unwired: 13 in, 1 out]
      }
      frame "Macro: Exit" {
        # "Exit Macro\n(This is called once, when the VI exits)"
        n154 = Unbundle By Name(w379) -> ("Core.Close Panel on Exit?"=w378:bool)
        n155 = Select(t="UI: Front Panel State >> Close\n", s=w378, f="") -> (s? t:f=w374:string)
        n156 = Concatenate Strings(w374, "Data: Cleanup\nExit") -> (w372:string)
        n157 = call "Enqueue Multiple States.vi"("State(s) at Front"=w372, "queue in"=w375) -> ()  [unwired: 13 in, 1 out]
      }
      frame "---------- Menu ----------" {
        # "Template Separator\n(You can make a copy of, or modify, this frame)"
        n158 = call "Enqueue Multiple States.vi"("queue in"=w381) -> ()  [unwired: 14 in, 1 out]
      }
      frame "Menu: Initialize" {
        n159 = Unbundle By Name(w385) -> ("Core.Menu Ref"=w384:refnum<k9>)
        n160 = call "Easy XML Editor Menu.vi"("error in (no error)"=w387, "Menu Refnum In"=w384) -> ("error out"=w386:errorcluster)  [unwired: 8 in, 1 out]
      }
      frame "Menu: Activate" {
        n161 = case shown="\"XML_UseStoredResources\"" w389 {
          selector: w389 -> [_ w394 w397 w400 w403 w406 w409 w412]
          tunnel: [_ w393 w396 w399 w402 w405 w408 w411] -> w388
          frame Default {
          }
          frame "XML_UseVTT" {
            n162 = Format Into String(format string="Data: Update >> Use VTT?\nMenu: Refresh >> %s", w394) -> (resulting string=w393:string)  [unwired: 2 in, 1 out]
          }
          frame "XML_Update" {
            n163 = Format Into String(format string="Data: Source VI to Res Data\nMenu: Refresh >> %s", w397) -> (resulting string=w396:string)  [unwired: 2 in, 1 out]
          }
          frame "XML_Save" {
            n164 = Format Into String(format string="Data: Save VI from Res Data\nMenu: Refresh >> %s", w400) -> (resulting string=w399:string)  [unwired: 2 in, 1 out]
          }
          frame "XML_EditedVIResEdit" {
            n165 = Format Into String(format string="UI: Resource Editor\nMenu: Refresh >> %s", w403) -> (resulting string=w402:string)  [unwired: 2 in, 1 out]
          }
          frame "XML_EditedVIOpen" {
            n166 = Format Into String(format string="UI: Open Edited VI\nMenu: Refresh >> %s", w406) -> (resulting string=w405:string)  [unwired: 2 in, 1 out]
          }
          frame "XML_StoredResEdit" {
            n167 = Format Into String(format string="UI: Edit Stored Resources\nMenu: Refresh >> %s", w409) -> (resulting string=w408:string)  [unwired: 2 in, 1 out]
          }
          frame "XML_UseStoredResources" {
            n168 = Format Into String(format string="Data: Update >> Use Stored Resources?\nMenu: Refresh >> %s", w412) -> (resulting string=w411:string)  [unwired: 2 in, 1 out]
          }
        }
        n169 = call "Enqueue Multiple States.vi"("queue in"=w390, "State(s) at Back"=w388) -> ()  [unwired: 13 in, 1 out]
      }
      frame "Menu: Refresh" {
        n170 = Unbundle By Name(w418) -> ("Use Stored Resources?"=w414:bool, "Stored Resources"=w415:T2[], "Use VTT?"=w416:bool, "Core.Menu Ref"=w417:refnum<k9>)
        n171 = case shown="\"XML_Update\"" w421 {
          selector: w421 -> [w423 w432 _ _ _ _ _ w458]
          tunnel: w420 -> [_ w435 w439 w447 w452 w453 w454 w466]
          tunnel: [w422 w434 w438 w446 w452 w453 w454 w457] -> w419
          tunnel: w417 -> [_ w433 w436 w444 _ _ _ w459]
          tunnel: w416 -> [_ w431 _ _ _ _ _ _]
          tunnel: w415 -> [_ _ _ _ _ _ _ w456]
          tunnel: w414 -> [_ _ _ _ _ _ _ w455]
          frame Default {
            n172 = xnode "Error Ring"("parameter 0"=w423) -> ("error out"=w422:errorcluster)
          }
          frame "XML_UseVTT" {
            n173 = Set Menu Item Info(6:w431, 7:w432, 8:w435, 11:w433) -> (0:w434:errorcluster)  [unwired: 3 in, 1 out]
          }
          frame "XML_Update" {
            w441 = TRUE ("enabled")
            n174 = Set Menu Item Info(7:"XML_StoredResEdit", 8:w439, 9:w441, 11:w436) -> (0:w437:errorcluster, 3:w443:refnum<k9>)  [unwired: 3 in]
            n175 = Set Menu Item Info(7:"XML_Save", 8:w437, 9:w441, 11:w443) -> (0:w438:errorcluster)  [unwired: 3 in, 1 out]
          }
          frame "XML_Save" {
            w448 = TRUE ("enabled")
            n176 = Set Menu Item Info(7:"XML_EditedVIResEdit", 8:w447, 9:w448, 11:w444) -> (0:w445:errorcluster, 3:w451:refnum<k9>)  [unwired: 3 in]
            n177 = Set Menu Item Info(7:"XML_EditedVIOpen", 8:w445, 9:w448, 11:w451) -> (0:w446:errorcluster)  [unwired: 3 in, 1 out]
          }
          frame "XML_EditedVIResEdit" {
          }
          frame "XML_EditedVIOpen" {
          }
          frame "XML_StoredResEdit" {
          }
          frame "XML_UseStoredResources" {
            n178 = Array Size(array=w456) -> (size(s)=w463:i32)
            n179 = Greater Than 0?(x=w463) -> (x > 0?=w462:bool)
            n180 = Implies(1:w462, 2:w455) -> (0:w461:bool)
            n181 = Set Menu Item Info(6:w455, 7:w458, 8:w466, 11:w459) -> (0:w465:errorcluster, 3:w464:refnum<k9>)  [unwired: 3 in]
            n182 = Set Menu Item Info(7:"XML_Save" ("item tag"), 8:w465, 9:w461, 11:w464) -> (0:w457:errorcluster)  [unwired: 3 in, 1 out]
          }
        }
      }
    }
  }
  n183 = Merge Errors(w10, w11) -> (w9:errorcluster)
  n184 = Release Queue(queue=w8, error in (no error)=w9) -> (error out=w3:errorcluster)  [unwired: 1 in, 2 out]
  n185 = Unregister For Events(event registration refnum=w2, error in=w3) -> ()  [unwired: 1 out]
